vi "get_MessageAndLabels.vi"(0 "HB_Dialog in":refnum<class "HB_Dialog.lvclass">, 11 "error in (no error)":errorcluster) -> (4 "HB_Dialog out":refnum<class "HB_Dialog.lvclass">, 6 "Message":string, 8 "T button name":string, 10 "F button name":string, 15 "error out":errorcluster)   [LabVIEW 2009, in "HB_Inherance_Example.lvlib" / "HB_Dialog.lvclass"]
doc: "Read attribute data."
uses:
  HB_Dialog.lvclass
  HB_Dialog.lvclass/HB_Dialog.ctl
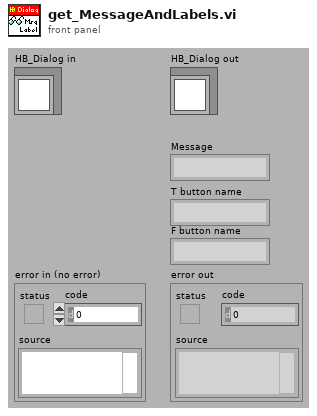
[diagram p1: front panel]
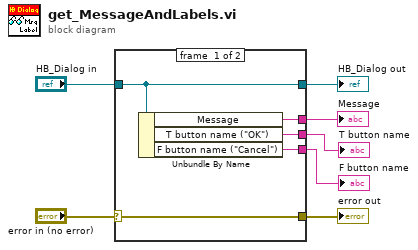
[diagram p0: block diagram]
diagram:
  n1 = case shown="No Error" "error in (no error)" {
    selector: "error in (no error)" -> [w12 w13]
    tunnel: [w12 w13] -> w6
    tunnel: [w11 w14] -> w4
    tunnel: "HB_Dialog in" -> [w11 w14]
    tunnel: [w8 _] -> w3
    tunnel: [w10 _] -> w2
    tunnel: [w9 _] -> w1
    frame #0 {
      n2 = Unbundle By Name(w11) -> ("Message"=w8:string, "T button name (\"OK\")"=w10:string, "F button name (\"Cancel\")"=w9:string)
    }
    frame #1 {
    }
  }
  "error out" <- w6
  "HB_Dialog out" <- w4
  "Message" <- w3
  "T button name" <- w2
  "F button name" <- w1
